vi "Get Pixel from Picture.vi"(8 "错误输入":errorcluster, 10 "Pos":T1, 11 "Picture in":picture) -> (0 "错误输出":errorcluster, 2 "Color":u32(colorbox), 3 "Picture out":picture)   [LabVIEW 2011]
uses:
  <vilib>/Utility/miscctls.llb/LVPoint32TypeDef.ctl
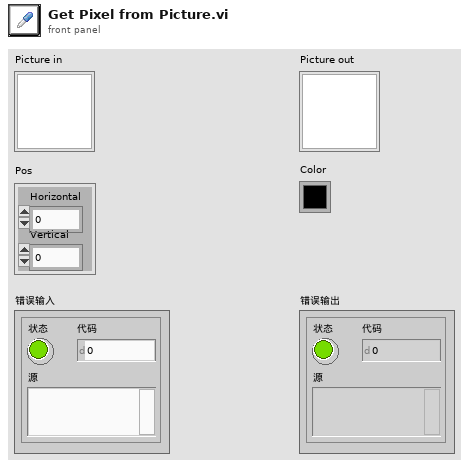
[diagram p1: front panel]
types:
  T1 = typedef "LVPoint32TypeDef.ctl" = cluster{"Horizontal":i32, "Vertical":i32}
  T2 = typedef "imagedata.ctl" = cluster{"image type":i32, "image depth":i32, "image":u8[], "mask":u8[], "colors":u32[], "Rectangle":cluster{"left":i16, "top":i16, "right":i16, "bottom":i16}}
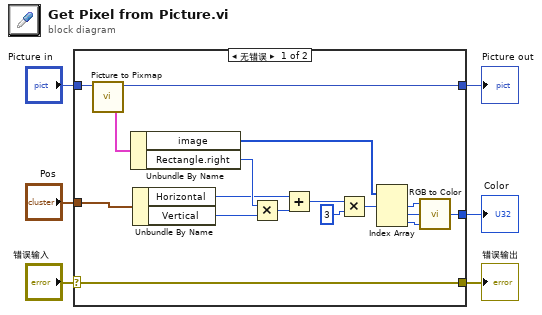
[diagram p0: block diagram]
diagram:
  n1 = case shown="无错误" "错误输入" {
    selector: "错误输入" -> [w23 w24]
    tunnel: [w23 w24] -> w5
    tunnel: "Picture in" -> [w22 _]
    tunnel: [w21 _] -> w3
    tunnel: "Pos" -> [w20 _]
    tunnel: [w7 _] -> w1
    frame No Error {
      n2 = call <vilib>:"Picture to Pixmap.vi"("picture"=w22) -> ("image data"=w19:T2, "new picture"=w21:picture)  [unwired: 9 in]
      n3 = Unbundle By Name(w19) -> ("image"=w11:u8[], "Rectangle.right"=w17:i16)
      n4 = Unbundle By Name(w20) -> ("Horizontal"=w15:i32, "Vertical"=w18:i32)
      n5 = Multiply(x=w17, y=w18) -> (x*y=w16:i32)
      n6 = Add(x=w15, y=w16) -> (x+y=w14:i32)
      n7 = Multiply(x=w14, y=3) -> (x*y=w12:i32)
      n8 = Index Array(array=w11, index #1=w12) -> (element #1=w10:u8, element #2=w9:u8, element #3=w8:u8)  [unwired: 2 in]
      n9 = call <vilib>:"RGB to Color.vi"("B"=w8, "G"=w9, "R"=w10) -> ("Color"=w7:u32)
    }
    frame Error {
    }
  }
  "错误输出" <- w5
  "Picture out" <- w3
  "Color" <- w1
